vi "GDX-ACC.vi"() -> ()   [LabVIEW 2019]
panel:
  out "Z-axis Standard Gravity (g)":dbl format="%.2g"
  out "Y-axis Standard Gravity (g)":dbl format="%.2g"
  out "X-axis Standard Gravity (g)":dbl format="%.2g"
  in  "Sample Rate (samples/sec)":dbl=50.0
  out "Waveform Chart":dbl[][](graph)
  in  "stop":bool
  out "error out":errorcluster
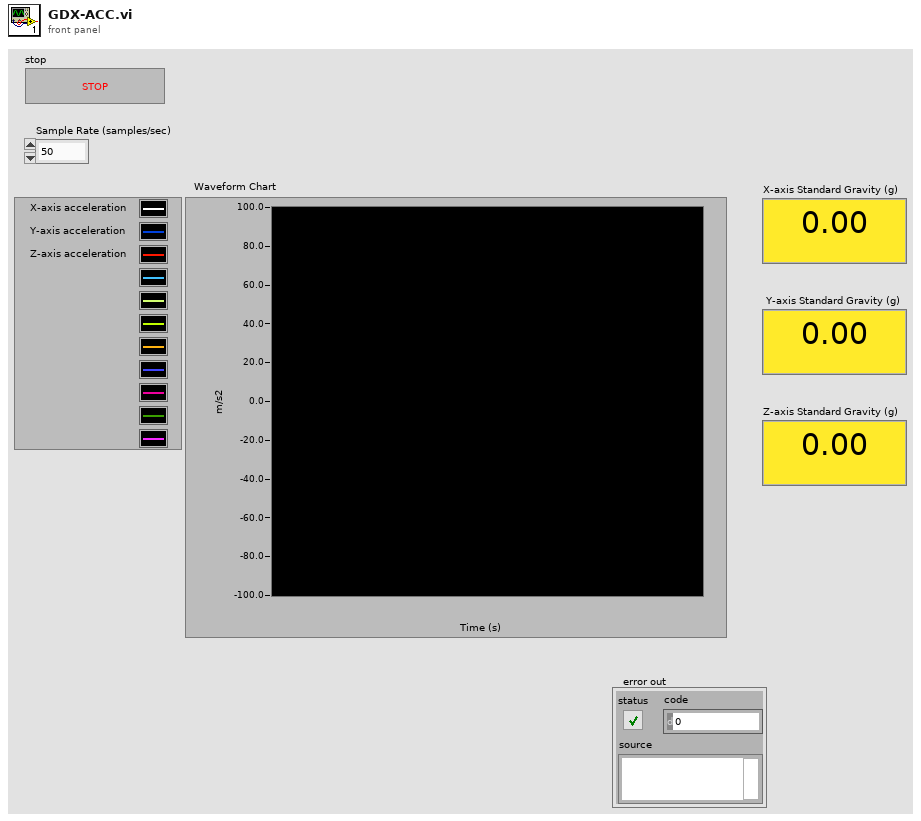
[diagram p1: front panel]
types:
  T1 = enum16{"Activate from Dialog Popup", "Activate All Channels", "Input On/Off Array", "Input Channel  Mask", "Burn Sensor Default Channels"}
  T2 = enum16{"Open from Dialog Popup", "Open all Available Devices", "Input Device Names"}
  T3 = enum16{"Set Rate from Dialog Popup", "Default 1 Sample/Sec", "Input Sample Rate"}
  T4 = typedef "D2PIO_D2PIOCluster.ctl" = cluster{"Library Handle":i64, "Device List Handle":i64, "BT Device Handles":i64[], "USB Device Handles":i64[], "BT+USB Device Handles":i64[], "Measurement Tick":dbl[], "Ch Availability Mask":u32[]}
  T5 = typedef "D2PIO_ChannelInfoCluster.ctl" = cluster{"Channel":i8, "Ch is Active":bool, "Channel ID":u32, "Channel Description":string, "Channel Unit":string}[]
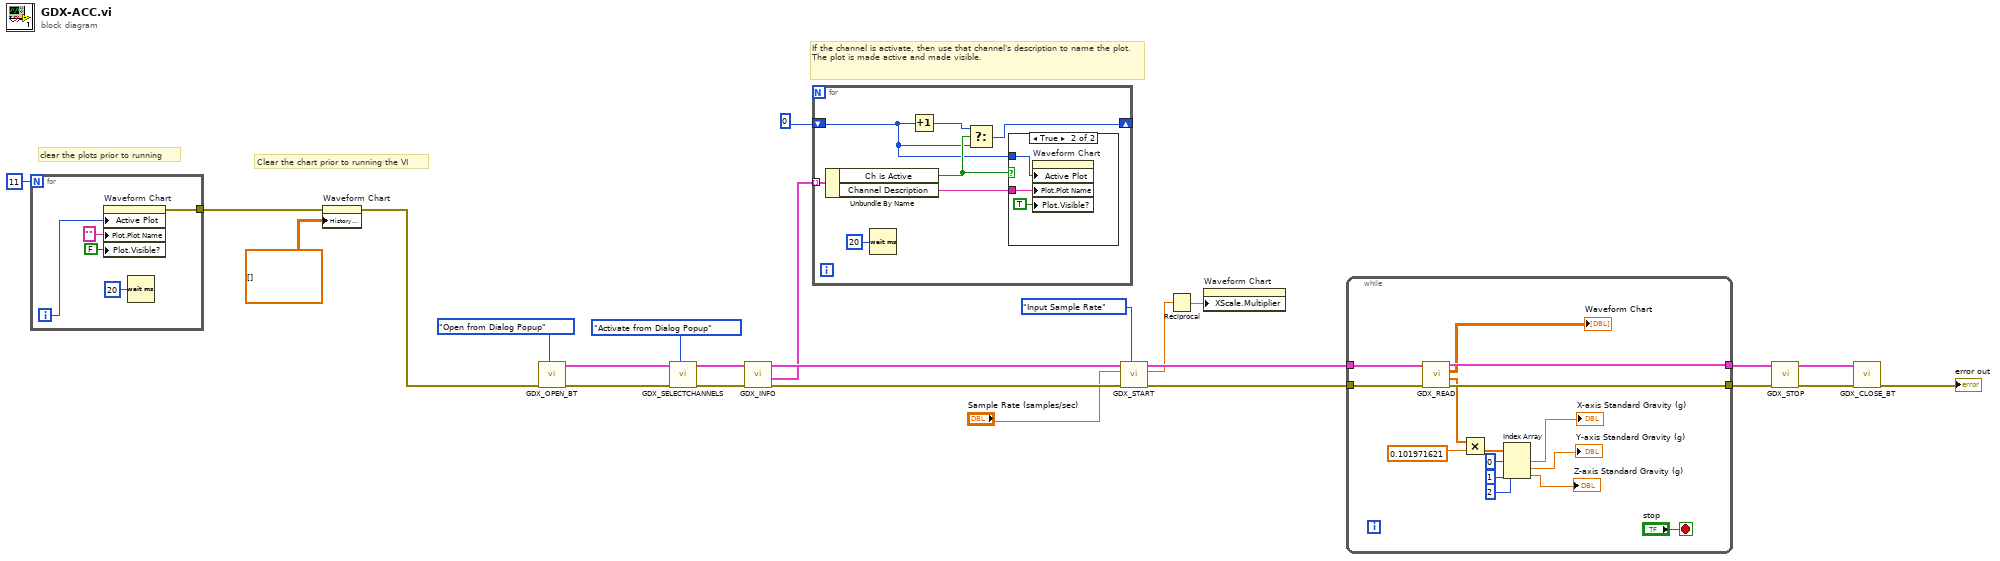
[diagram p0: block diagram]
diagram:
  # "If the channel is activate, then use that channel's description to name the plot. The plot is made active and made visible."
  # "clear the plots prior to running"
  # "Clear the chart prior to running the VI"
  n1 = for {
    N: 11 -> [_]
    tunnel: [w26] -> w3
    i -> [w28]
    n2 = property on="Waveform Chart" class="WFChart (strict)"("Active Plot"=w28, "Plot.Plot Name"="", "Plot.Visible?"=FALSE ("Plot.Visible")) -> (error out=w26:errorcluster)  [unwired: 2 in, 1 out]
    n3 = Wait (ms)(milliseconds to wait=u32 20) -> ()  [unwired: 1 out]
  }
  n4 = property on="Waveform Chart" class="WFChart (strict)"(error in=w3, "History Data"=dbl[][] [] ("Waveform Chart")) -> (error out=w8:errorcluster)  [unwired: 1 in, 1 out]
  n5 = call <vilib>:"GDX_OPEN_BT.vi"("Enum"=T2."Open from Dialog Popup", "error in (no error)"=w8) -> ("error out"=w18:errorcluster, "D2PIO Cluster Out"=w19:T4)  [unwired: 8 in]
  n6 = call <vilib>:"GDX_SELECTCHANNELS.vi"("Enum"=T1."Activate from Dialog Popup", "error in (no error)"=w18, "D2PIO Cluster In"=w19) -> ("error out"=w13:errorcluster, "D2PIO Cluster Out"=w14:T4)  [unwired: 7 in]
  n7 = call <vilib>:"GDX_INFO.vi"("error in (no error)"=w13, "D2PIO Cluster In"=w14) -> ("error out"=w11:errorcluster, "Array of Channel Info Cluster"=w10:T5, "D2PIO Cluster Out"=w12:T4)  [unwired: 4 in, 3 out]
  n8 = for {
    tunnel: w10 -> [w37] mode=indexing
    shift-right: [w33] -> _
    shift-left: u32 0 ("Active Plot") -> [w31]
    n9 = Unbundle By Name(w37) -> ("Ch is Active"=w34:bool, "Channel Description"=w36:string)
    n10 = Wait (ms)(milliseconds to wait=u32 20) -> ()  [unwired: 1 out]
    n11 = Increment(x=w31) -> (x+1=w32:u32)
    n12 = Select(t=w32, s=w34, f=w31) -> (s? t:f=w33:u32)
    n13 = case shown="True" w34 {
      tunnel: w36 -> [_ w40]
      tunnel: w31 -> [_ w39]
      frame False {
      }
      frame True {
        n14 = property on="Waveform Chart" class="WFChart (strict)"("Active Plot"=w39, "Plot.Plot Name"=w40, "Plot.Visible?"=TRUE ("Plot.Visible")) -> ()  [unwired: 2 in, 2 out]
      }
    }
  }
  n15 = call <vilib>:"GDX_START.vi"("Enum"=T3."Input Sample Rate", "error in (no error)"=w11, "Sample Rate (samples/sec)"="Sample Rate (samples/sec)", "D2PIO Cluster In"=w12) -> ("error out"=w25:errorcluster, "Actual Sample Rate"=w16:dbl, "D2PIO Cluster Out"=w24:T4)  [unwired: 4 in, 1 out]
  n16 = Reciprocal(x=w16) -> (1/x=w15:dbl)
  n17 = property on="Waveform Chart" class="WFChart (strict)"("XScale.Multiplier"=w15) -> ()  [unwired: 2 in, 2 out]
  n18 = while {
    tunnel: w25 -> [w55]
    tunnel: w24 -> [w53]
    tunnel: [w52] -> w23
    tunnel: [w51] -> w17
    stop <- "stop" stop-if-true
    n19 = call <vilib>:"GDX_READ.vi"("error in (no error)"=w55, "D2PIO Cluster In"=w53) -> ("error out"=w51:errorcluster, "Data"=w46:dbl[], "Waveform Chart Data"=→"Waveform Chart":dbl[][], "D2PIO Cluster Out"=w52:T4)  [unwired: 4 in, 2 out]
    n20 = Multiply(x=w46, y=0.101971621) -> (x*y=w44:dbl[])
    n21 = Index Array(array=w44, index #1=0 ("index"), index #2=1 ("index"), index #3=2 ("index")) -> (element #1=→"X-axis Standard Gravity (g)":dbl, element #2=→"Y-axis Standard Gravity (g)":dbl, element #3=→"Z-axis Standard Gravity (g)":dbl)
  }
  n22 = call <vilib>:"GDX_STOP.vi"("error in (no error)"=w17, "D2PIO Cluster In"=w23) -> ("error out"=w21:errorcluster, "D2PIO Cluster Out"=w22:T4)  [unwired: 8 in]
  n23 = call <vilib>:"GDX_CLOSE_BT.vi"("error in (no error)"=w21, "D2PIO Cluster In"=w22) -> ("error out"=→"error out":errorcluster)  [unwired: 8 in, 1 out]
